vi "autofocus calibrate.vi"(8 "Error In":errorcluster, 11 "Handle":i32) -> (0 "Error Out":errorcluster, 1 "Cal. Curve (current z)":cluster{ext[], dbl[]}, 2 "Intensity OK":bool=TRUE, 3 "Cal. curve":cluster{ext[], dbl[]})   [LabVIEW 2014]
uses:
  Shutter Control/Shutter SubVIs/ctts/user event shutter global.ctl
  Stage Control/Stage SubVIs/ctts/move stage.ctl
  autofocus-globals.vi
  TIRF/tirf-lock-globals.vi
panel:
  out "XY Position":cluster{"Y":dbl[], "Y":dbl[]}[](graph)=[{"Y"=[30.68], "Y"=[27.36]}]
  out "Power Intensity":dbl(graph)
  out "Intensity 2":cluster{"X position":dbl, "Y position":dbl}(graph)
  out "Calibration curve":cluster{ext[], dbl[]}(graph)
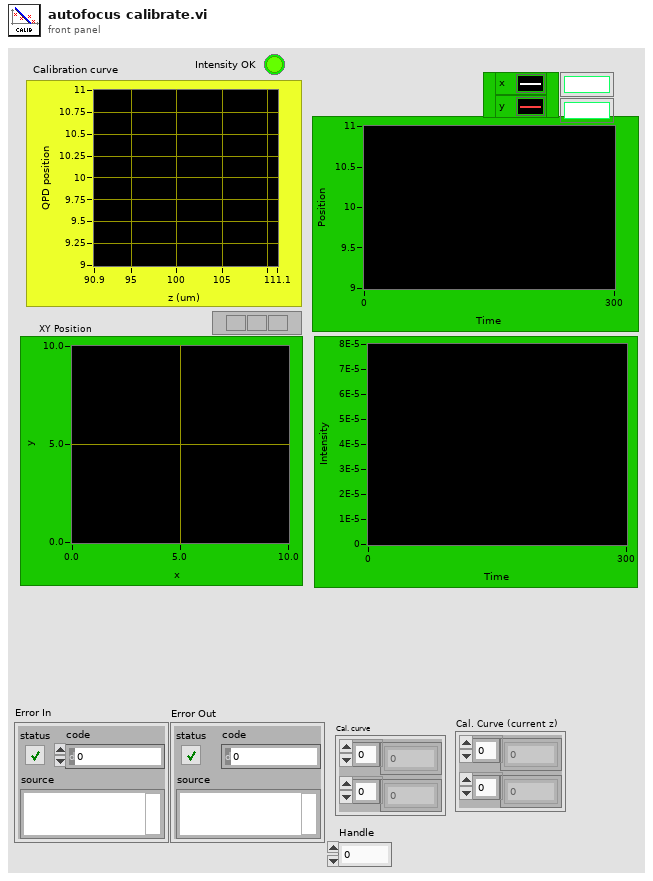
[diagram p1: front panel]
types:
  T1 = enum32{"Invalid", "Standard", "Closed", "Hidden", "Minimized", "Maximized"}
  T2 = enum32{"No Selection", "GFP", "Cy3 Long \nPass", "Cy3", "Cy5", "Off", "IR"}
  T3 = typedef "user event shutter global.ctl" = cluster{"Camera Shutter":bool, "Laser Shutter":enum32{"No Selection", "GFP", "Cy3 Long \nPass", "Cy3", "Cy5", "Off", "IR"}}
  T4 = typedef "move stage.ctl" = cluster{"dx (um) (0 -> ignore)":ext, "dy (um) (0 -> ignore)":ext, "dz (um) (0 -> ignore)":ext, "Re-center x,y":bool, "Re-center z":bool, "x (um) (-1 -> ignore)":dbl, "y (um) (-1 -> ignore)":dbl, "z (um) (-1 -> ignore)":dbl, "Move to Next Field":bool}
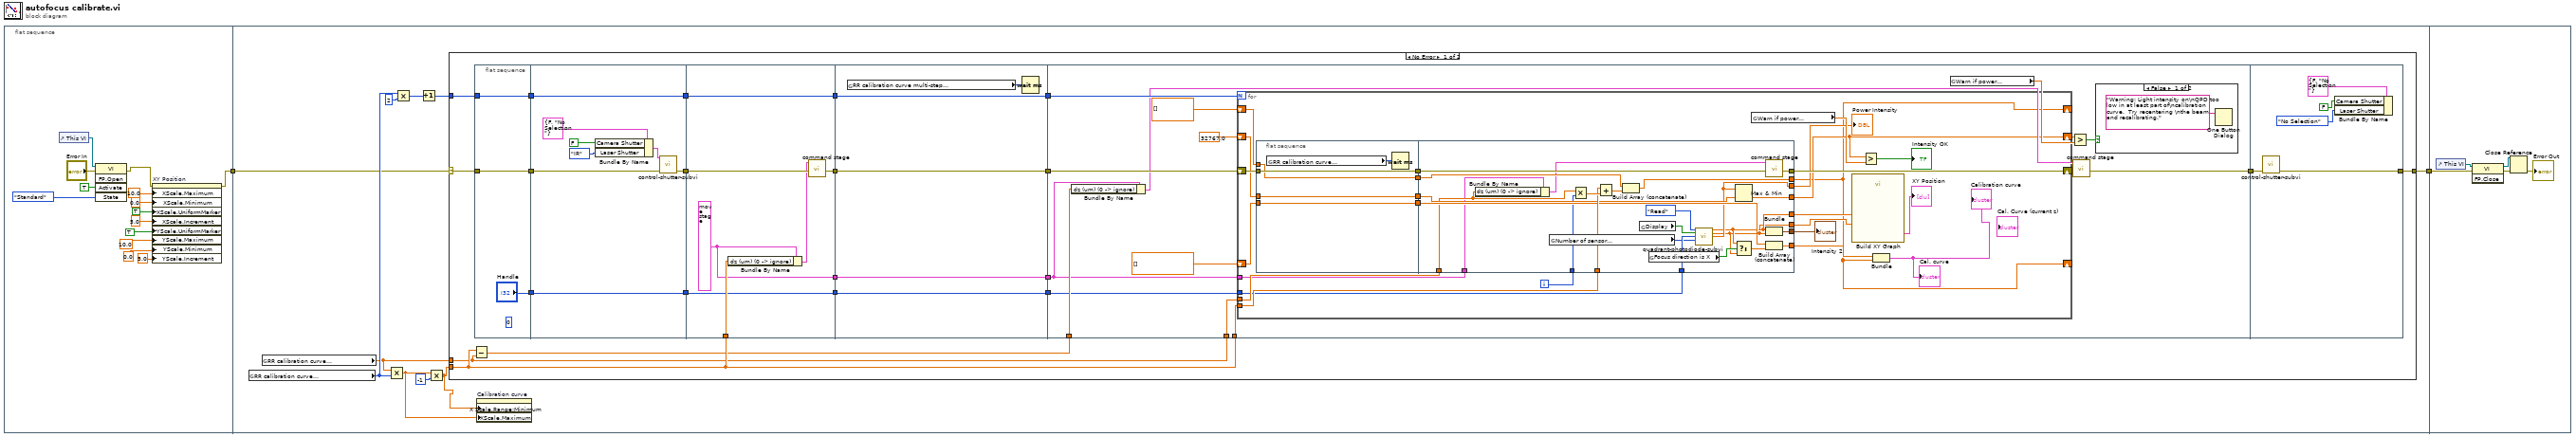
[diagram p0: block diagram]
diagram:
  n1 = flat-sequence {
    tunnel: [w3] -> w1
    tunnel: [w20] -> w2
    tunnel: w1 -> [w19]
    tunnel: w2 -> [w150]
    frame #0 {
      n2 = control-ref of="This VI"() -> (w16:refnum<vi>)
      n3 = invoke class="VI" method="FP.Open"(reference=w16, error in="Error In", "Activate"=TRUE ("Activate?"), "State"=T1."Standard") -> (error out=w4:errorcluster)  [unwired: 1 in, 4 out]
      n4 = property on="XY Position" class="XYGraph (strict)"(error in=w4, "XScale.Maximum"=10.0 ("X Scale.Range:Maximum"), "XScale.Minimum"=0.0 ("X Scale.Range:Minimum"), "XScale.UniformMarker"=TRUE ("X Scale.Uniform Marker Spacing?"), "XScale.Increment"=5.0 ("X Scale.Range:Increment"), "YScale.UniformMarker"=TRUE ("Y Scale.Uniform Marker Spacing?"), "YScale.Maximum"=10.0 ("Y Scale.Range:Maximum"), "YScale.Minimum"=0.0 ("Y Scale.Range:Minimum"), "YScale.Increment"=5.0 ("Y Scale.Range:Increment")) -> (error out=w3:errorcluster)  [unwired: 1 in, 1 out]
    }
    frame #1 {
      n5 = global read "autofocus-globals.vi" "RR calibration curve\nhalf-width  (steps)"() -> (w24:u32)
      n6 = global read "autofocus-globals.vi" "RR calibration curve\nstep size (um)"() -> (w21:ext)
      n7 = Multiply(x=w21, y=w24) -> (x*y=w18:ext)
      n8 = Multiply(x=w24, y=2) -> (x*y=w23:u32)
      n9 = Increment(x=w23) -> (x+1=w22:u32)
      n10 = Multiply(x=w18, y=-1) -> (x*y=w17:ext)
      n11 = case shown="No Error" w19 {
        selector: w19 -> [w27 w148]
        tunnel: [w28 w148] -> w20
        tunnel: w17 -> [w36 _]
        tunnel: w22 -> [w47 _]
        tunnel: w21 -> [w35 _]
        frame No Error {
          n12 = Subtract(x=w36, y=w35) -> (x-y=w34:ext)
          n13 = flat-sequence {
            tunnel: w47 -> [w50]
            tunnel: [w48] -> w46
            tunnel: [w50] -> w40
            tunnel: ["Handle"] -> w29
            tunnel: w27 -> [w48]
            tunnel: w46 -> [w56]
            tunnel: [w55] -> w45
            tunnel: [w58] -> w41
            tunnel: w40 -> [w58]
            tunnel: [w57] -> w30
            tunnel: w29 -> [w57]
            tunnel: w45 -> [w65]
            tunnel: w36 -> [w63]
            tunnel: [w64] -> w44
            tunnel: [w61] -> w43
            tunnel: [w60] -> w42
            tunnel: w41 -> [w60]
            tunnel: [w59] -> w31
            tunnel: w30 -> [w59]
            tunnel: w44 -> [w70]
            tunnel: w43 -> [w69]
            tunnel: w42 -> [w67]
            tunnel: [w70] -> w39
            tunnel: [w69] -> w38
            tunnel: [w67] -> w37
            tunnel: [w66] -> w32
            tunnel: w31 -> [w66]
            tunnel: w39 -> [w85]
            tunnel: w38 -> [w76]
            tunnel: w37 -> [w86]
            tunnel: w36 -> [w81]
            tunnel: w35 -> [w80]
            tunnel: w34 -> [w78]
            tunnel: [w75] -> w33
            tunnel: w32 -> [w71]
            tunnel: w33 -> [w147]
            tunnel: [w146] -> w28
            frame #0 {
              (unwired) 0
            }
            frame #1 {
              n14 = Bundle By Name(cluster=T3 {"Camera Shutter"=FALSE, "Laser Shutter"=enum."No Selection"} ("Shutter Control"), "Camera Shutter"=FALSE, "Laser Shutter"=T2."IR") -> (w51:T3)
              n15 = call "control-shutter-subvi.vi"("Error In"=w56, "Shutter Control"=w51) -> ("Error Out"=w55:errorcluster)  [unwired: 9 in]
            }
            frame #2 {
              w61 = T4 {"dx (um) (0 -> ignore)"=0.0, "dy (um) (0 -> ignore)"=0.0, "dz (um) (0 -> ignore)"=0.0, "Re-center x,y"=FALSE, "Re-center z"=FALSE, "x (um) (-1 -> ignore)"=-1.0, "y (um) (-1 -> ignore)"=-1.0, "z (um) (-1 -> ignore)"=-1.0, "Move to Next Field"=FALSE} ("Command Stage")
              n16 = Bundle By Name(cluster=w61, "dz (um) (0 -> ignore)"=w63) -> (w62:T4)
              n17 = call "command stage.vi"("Error In"=w65, "Command Stage"=w62) -> ("Error Out"=w64:errorcluster)  [unwired: 9 in]
            }
            frame #3 {
              n18 = global read "autofocus-globals.vi" "RR calibration curve multi-step\nadd'l settle time (ms)"() -> (w68:u16)
              n19 = Wait (ms)(milliseconds to wait=w68) -> ()  [unwired: 1 out]
            }
            frame #4 {
              n20 = Bundle By Name(cluster=w76, "dz (um) (0 -> ignore)"=w78) -> (w77:T4)
              n21 = for {
                N: w86 -> [_]
                shift-right: [w104] -> w79
                shift-left: w85 -> [w112]
                shift-right: [w97] -> w74
                shift-left: 32767.0 -> [w108]
                shift-right: [w90] -> _
                shift-left: dbl[] [] ("z (um)") -> [w109]
                shift-right: [w89] -> _
                shift-left: dbl[] [] ("QPD position") -> [w110]
                tunnel: w81 -> [w103]
                tunnel: w80 -> [w101]
                tunnel: w76 -> [w100]
                tunnel: w71 -> [w96]
                i -> [w102]
                n22 = flat-sequence {
                  tunnel: w112 -> [w116]
                  tunnel: [w116] -> w111
                  tunnel: w110 -> [w115]
                  tunnel: w109 -> [w114]
                  tunnel: w108 -> [w113]
                  tunnel: [w115] -> w107
                  tunnel: [w114] -> w106
                  tunnel: [w113] -> w105
                  tunnel: w111 -> [w124]
                  tunnel: w107 -> [w135]
                  tunnel: w106 -> [w136]
                  tunnel: w105 -> [w138]
                  tunnel: [w140] -> w104
                  tunnel: w103 -> [w139]
                  tunnel: [w137] -> w97
                  tunnel: [w133] -> w89
                  tunnel: w102 -> [w132]
                  tunnel: w101 -> [w131]
                  tunnel: w100 -> [w130]
                  tunnel: [w128] -> w90
                  tunnel: w96 -> [w126]
                  tunnel: [w121] -> w95
                  tunnel: [w120] -> w94
                  tunnel: [w119] -> w92
                  tunnel: [w118] -> w91
                  frame #0 {
                    n23 = global read "autofocus-globals.vi" "RR calibration curve\nsettle time (ms)"() -> (w117:u32)
                    n24 = Wait (ms)(milliseconds to wait=w117) -> ()  [unwired: 1 out]
                  }
                  frame #1 {
                    n25 = Bundle By Name(cluster=w130, "dz (um) (0 -> ignore)"=w131) -> (w122:T4)
                    n26 = global read "autofocus-globals.vi" "Number of sensor\nreadings to average"() -> (w125:i32)
                    n27 = Multiply(x=w131, y=w132) -> (x*y=w142:ext)
                    n28 = Add(x=w139, y=w142) -> (x+y=w141:ext)
                    n29 = Build Array (concatenate)(w136, w141) -> (w128:ext[])
                    n30 = global read "tirf-lock-globals.vi" "Display"() -> (w123:bool)
                    n31 = global read "autofocus-globals.vi" "Focus direction is X"() -> (w129:bool)
                    n32 = call "quadrant-photodiode-subvi.vi"("Mode"=enum16{"Start", "Read", "End"}."Read", "Display"=w123, "Handle"=w126, "Averages"=w125) -> ("coerced(x)"=w119:dbl, "coerced(y)"=w118:dbl, "Power (mw)"=w120:dbl)  [unwired: 9 in]
                    n33 = Select(t=w119, s=w129, f=w118) -> (s? t:f=w134:dbl)
                    n34 = Max & Min(x=w120, y=w138) -> (min(x,y)=w137:dbl)  [unwired: 1 out]
                    n35 = call "command stage.vi"("Error In"=w124, "Command Stage"=w122) -> ("Error Out"=w140:errorcluster)  [unwired: 9 in]
                    n36 = Bundle("coerced(x)"=w119, "coerced(y)"=w118) -> (w121:cluster{"coerced(x)":dbl, "coerced(y)":dbl})  [unwired: 1 in]
                    n37 = Build Array (concatenate)(w135, w134) -> (w133:dbl[])
                  }
                }
                n38 = global read "autofocus-globals.vi" "Warn if power \nless than"() -> (w98:dbl)
                n39 = call "Build XY Graph"("Y Input"=w91, "X Input"=w92) -> ("XY Graph"=→"XY Position":cluster{"Y":dbl[], "Y":dbl[]}[])  [unwired: 3 in, 6 out]
                n40 = Greater?(x=w97, y=w98) -> (0:→"Intensity OK":bool)
                n41 = Bundle(w90, w89) -> (→"Cal. curve" →"Calibration curve":cluster{ext[], dbl[]})  [unwired: 1 in]
                "Intensity 2" <- w95
                "Power Intensity" <- w94
              }
              n42 = global read "autofocus-globals.vi" "Warn if power \nless than"() -> (w73:dbl)
              n43 = Greater?(x=w74, y=w73) -> (0:w72:bool)
              n44 = call "command stage.vi"("Error In"=w79, "Command Stage"=w77) -> ("Error Out"=w75:errorcluster)  [unwired: 9 in]
              n45 = case shown="False" w72 {
                frame False {
                  n46 = One Button Dialog(message="Warning: Light intensity on\nQPD too low in at least part of\ncalibration curve.  Try recentering \nthe beam and recalibrating.") -> ()  [unwired: 2 out]
                }
                frame True {
                }
              }
            }
            frame #5 {
              n47 = call "control-shutter-subvi.vi"("Error In"=w147) -> ("Error Out"=w146:errorcluster)  [unwired: 10 in]
              n48 = Bundle By Name(cluster=T3 {"Camera Shutter"=FALSE, "Laser Shutter"=enum."No Selection"} ("Shutter Control"), "Camera Shutter"=FALSE, "Laser Shutter"=T2."No Selection") -> ()  [unwired: 1 out]
            }
          }
        }
        frame Error {
        }
      }
      n49 = property on="Calibration curve" class="XYGraph (strict)"("X Scale.Range:Minimum"=w17, "XScale.Maximum"=w18) -> ()  [unwired: 2 in, 2 out]
    }
    frame #2 {
      n50 = control-ref of="This VI"() -> (w149:refnum<vi>)
      n51 = invoke class="VI" method="FP.Close"(reference=w149, error in=w150) -> (reference out=w153:refnum<vi>, error out=w152:errorcluster)  [unwired: 1 in, 1 out]
      n52 = Close Reference(reference=w153, error in (no error)=w152) -> (error out=→"Error Out":errorcluster)
    }
  }
